vi "Title_Data_save.vi"(6 "ErrorIndex":i32, 8 "Data in":T1, 11 "AllControls In":T2) -> (2 "数组":string[](array[string]))   [LabVIEW 2017]
uses:
  Ctrls/AllControls.ctl
  Ctrls/CSV_Data.ctl
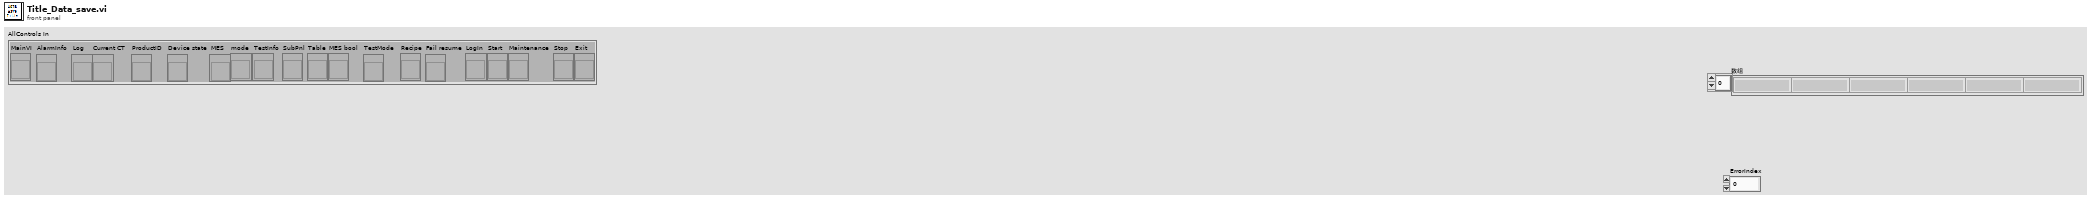
[diagram p1: front panel]
types:
  T1 = typedef "CSV_Data.ctl" = cluster{"Version":cluster{"SC_Version":string, "VP_Version":string}, "SN":string, "Table":string[][], "Count":cluster{"Total":i32, "OK":i32, "NG":i32, "Yield":dbl}, "Start Time":timestamp, "daemon reference":refnum<k5>, "CT":dbl, "Config":string[][], "OK/NG":bool, "Station ID":string, "MES DDM SN":string, "MES PCBA SN":string, "Retest":string, "Lux":string, "VOT":cluster{"Initial brightness":string, "Mean uniformity":string, "Uniformity_Deviation":string, "Adjusted brightness":string, "Mean_Adjusted":string, "Deviation_Adjusted":string, "Reflection":string, "Result":bool}, "SKU":string, "Plate_Diameter":string, "Alarm":string}
  T2 = typedef "AllControls.ctl" = cluster{"MainVI":refnum<vi>, "AlarmInfo":refnum<vi>, "Log":refnum<vi>, "Current CT":refnum<vi>, "ProductID":refnum<vi>, "Device state":refnum<vi>, "MES":refnum<vi>, "mode":refnum<vi>, "TestInfo":refnum<vi>, "SubPnl":refnum<vi>, "Table":refnum<vi>, "MES bool":refnum<vi>, "TestMode":refnum<vi>, "Recipe":refnum<vi>, "Fail resume":refnum<vi>, "LogIn":refnum<vi>, "Start":refnum<vi>, "Maintenance":refnum<vi>, "Stop":refnum<vi>, "Exit":refnum<vi>}
  T3 = typedef "HD Config.ctl" = cluster{" PC":cluster{"PC Address":u8[], "PC Port":i32}, "FCO":cluster{"COM":refnum<visa-resource-name>, "Baudrate":u32}, "DC Power ":cluster{"COM":refnum<visa-resource-name>, "Baudrate":u32}, "PW3336":cluster{"COM":refnum<visa-resource-name>, "Baudrate":u32}, "Lefoo":cluster{"COM":refnum<visa-resource-name>, "Baudrate":u32}, "Tempt&Hum":cluster{"COM":refnum<visa-resource-name>, "Baudrate":u32}, "DIPC":cluster{"COM":refnum<visa-resource-name>}, "Daemon":cluster{"IP Address":string, "Port":u16, "Retry":u16}, "NFC_Cmd":cluster{"COM":refnum<visa-resource-name>, "Baudrate":u32}, "Fail_resume_mode":bool, "GRR":bool, "NFC _Serial":cluster{"COM":refnum<visa-resource-name>, "Baudrate":u32}}
  T4 = typedef "TesterInfo.ctl" = cluster{"Station Name":string, "Station Code":string, "ES NO.":string, "Tester ID":string, "PassMark Revision":string, "Rig ID":string, "682_Tool_Repeat":string, "Project Name":string, "FFTesterPath":path, "Enable_User":bool, "Mode":enum16{"682"}, "Fail_resume_mode":bool}
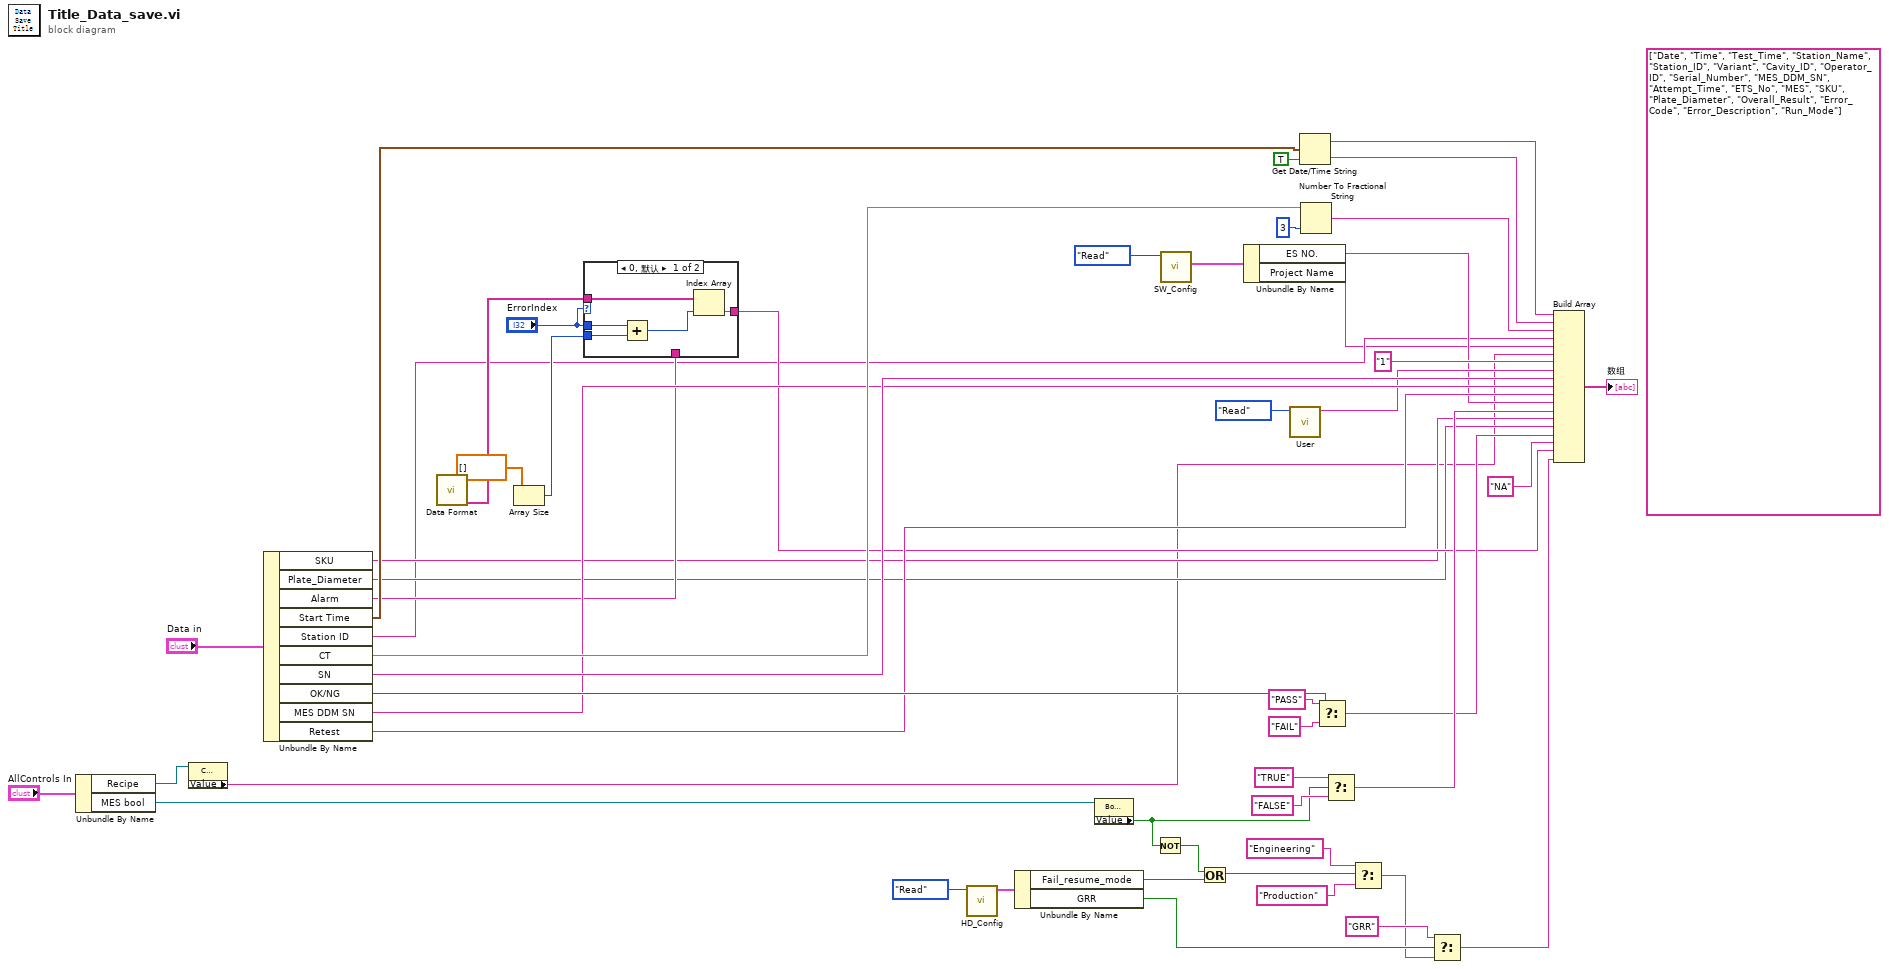
[diagram p0: block diagram]
diagram:
  (unwired) string[] ["Date", "Time", "Test_Time", "Station_Name", "Station_ID", "Variant", "Cavity_ID", "Operator_ID", "Serial_Number", "MES_DDM_SN", "Attempt_Time", "ETS_No", "MES", "SKU", "Plate_Diameter", "Overall_Result", "Error_Code", "Error_Description", "Run_Mode"]
  n1 = Unbundle By Name("AllControls In") -> ("Recipe"=w14:refnum<vi>, "MES bool"=w37:refnum<vi>)
  n2 = property class="CmbBox"(reference=w14) -> ("Value"=w4:string)  [unwired: 1 in, 2 out]
  n3 = Unbundle By Name("Data in") -> ("SKU"=w6:string, "Plate_Diameter"=w5:string, "Alarm"=w7:string, "Start Time"=w11:timestamp, "Station ID"=w3:string, "CT"=w39:dbl, "SN"=w47:string, "OK/NG"=w35:bool, "MES DDM SN"=w25:string, "Retest"=w20:string)
  n4 = call "Data Format.vi"() -> ("title"=w13:string[])  [unwired: 10 in, 1 out]
  n5 = Array Size(array=dbl[] []) -> (size(s)=w8:i32)
  n6 = case shown="0, 默认" "ErrorIndex" {
    tunnel: w13 -> [w57 _]
    tunnel: "ErrorIndex" -> [w56 _]
    tunnel: [w54 w58] -> w12
    tunnel: w8 -> [w53 _]
    tunnel: w7 -> [_ w58]
    frame 0, Default {
      n7 = Add(x=w56, y=w53) -> (x+y=w55:i32)
      n8 = Index Array(array=w57, index=w55) -> (element=w54:string)
    }
    frame -1 {
    }
  }
  n9 = call "HD_Config.vi"("Step"=enum16{"Initial", "Write", "Read"}."Read") -> ("HD Config out"=w33:T3)  [unwired: 9 in, 1 out]
  n10 = Unbundle By Name(w33) -> ("Fail_resume_mode"=w29:bool, "GRR"=w24:bool)
  n11 = property class="Bool (严格)"(reference=w37) -> ("Value"=w28:bool)  [unwired: 1 in, 2 out]
  n12 = Not(x=w28) -> (.not. x?=w26:bool)
  n13 = call "SW_Config.vi"("Step"=enum16{"Initial", "Write", "Read"}."Read") -> ("SW Config out"=w52:T4)  [unwired: 9 in, 1 out]
  n14 = Or(x=w26, y=w29) -> (x .or. y?=w27:bool)
  n15 = Unbundle By Name(w52) -> ("ES NO."=w17:string, "Project Name"=w2:string)
  n16 = call "User.vi"("Step"=enum16{"Initial", "Write", "Read"}."Read") -> ("User out"=w18:string)  [unwired: 9 in, 1 out]
  n17 = Get Date/Time String(seconds (now)=w11, want seconds? (F)=TRUE ("需要秒？(F)")) -> (date string=w41:string, time string=w42:string)  [unwired: 1 in]
  n18 = Number To Fractional String(number=w39, precision (6)=i16 3 ("精度(6)")) -> (F-format string=w44:string)  [unwired: 2 in]
  n19 = Select(t="PASS" ("真字符串"), s=w35, f="FAIL" ("假字符串")) -> (s? t:f=w15:string)
  n20 = Select(t="TRUE" ("真字符串"), s=w28, f="FALSE" ("假字符串")) -> (s? t:f=w16:string)
  n21 = Select(t="Engineering", s=w27, f="Production") -> (s? t:f=w22:string)
  n22 = Select(t="GRR", s=w24, f=w22) -> (s? t:f=w21:string)
  n23 = Build Array(w41, w42, w44, w3, w2, w4, "1" ("Cavity ID_L"), w18, w47, w25, w20, w17, w16, w6, w5, w15, "NA" ("element"), w12, w21) -> (→"数组":string[])
